vi "DrivetrainStateMachines(SubVI).vi"(4 "humanToSteady":bool, 5 "encoderSignalReceived?":bool, 6 "IMUtoSteady":bool, 7 "IMUSignalReceived?":bool, 9 "encoderToSteady":bool, 11 "humanSignalReceived?":bool) -> (3 "State Out":T1)   [LabVIEW 2017]
uses:
  Control 2.ctl
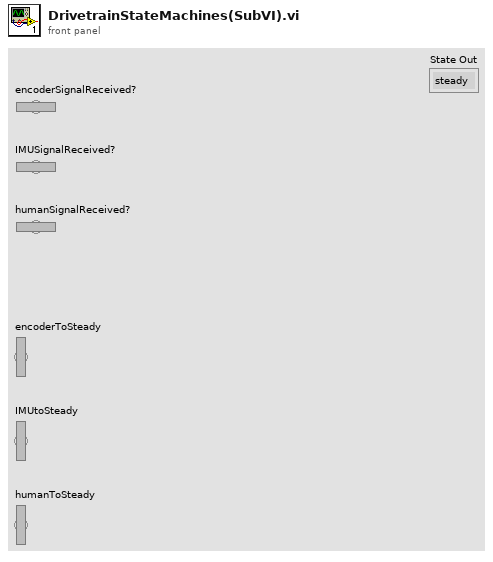
[diagram p1: front panel]
types:
  T1 = typedef "Control 2.ctl" = enum16{"steady", "driveByEncoder", "driveByIMU", "driveByHumans"}
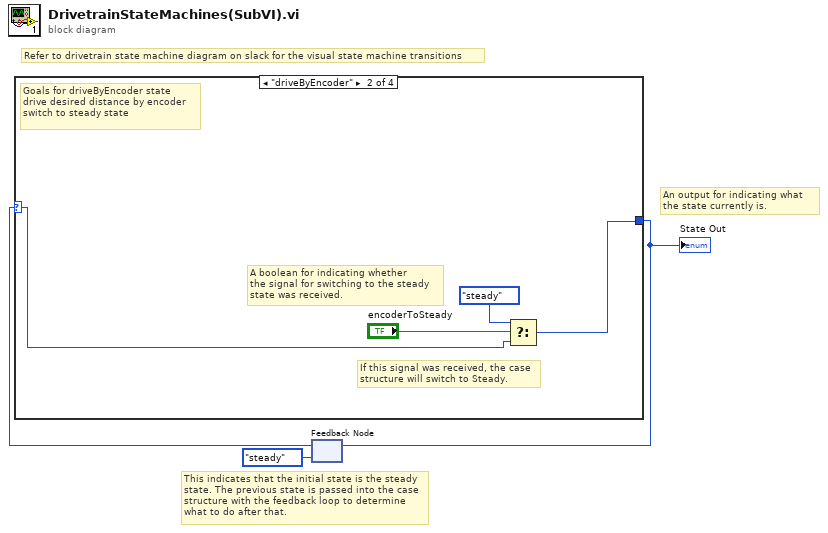
[diagram p0: block diagram]
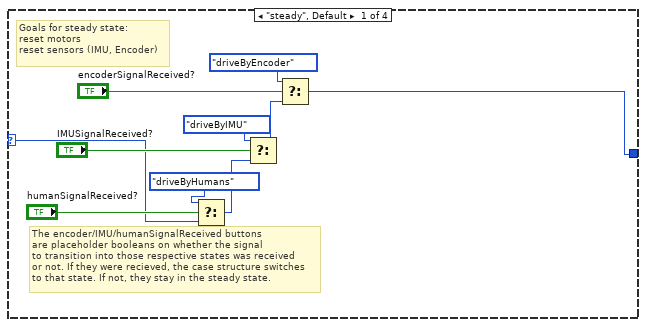
[diagram p2: hidden frame]
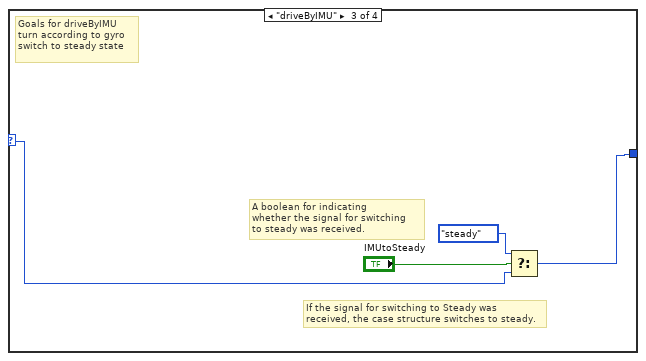
[diagram p3: hidden frame]
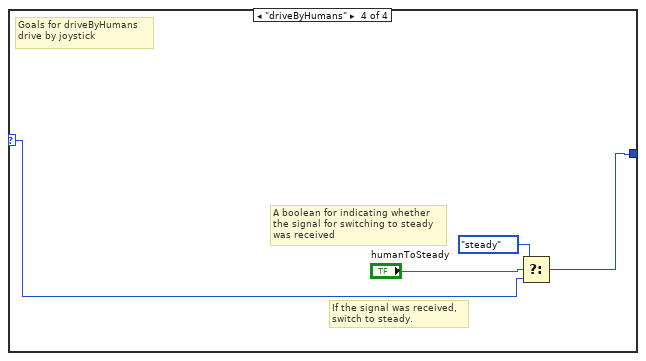
[diagram p4: hidden frame]
diagram:
  # "An output for indicating what\nthe state currently is."
  # "This indicates that the initial state is the steady\nstate. The previous state is passed into the case\nstructure with the feedback loop to determine\nwhat to do after that."
  # "Refer to drivetrain state machine diagram on slack for the visual state machine transitions"
  n1 = feedback #1(Control_2."steady") -> (w2:T1)
  n2 = case shown="\"driveByEncoder\"" w2 {
    selector: w2 -> [w4 w14 w18 w22]
    tunnel: [w7 w17 w20 w23] -> w3
    frame "steady", Default {
      # "The encoder/IMU/humanSignalReceived buttons\nare placeholder booleans on whether the signal\nto transition into those respective states was received\nor not. If they were recieved, the case structure switches\nto that state. If not, they stay in the steady state."
      # "Goals for steady state:\nreset motors\nreset sensors (IMU, Encoder)"
      n3 = Select(t=Control_2."driveByHumans", s="humanSignalReceived?", f=w4) -> (s? t:f=w6:T1)
      n4 = Select(t=Control_2."driveByIMU", s="IMUSignalReceived?", f=w6) -> (s? t:f=w5:T1)
      n5 = Select(t=Control_2."driveByEncoder", s="encoderSignalReceived?", f=w5) -> (s? t:f=w7:T1)
    }
    frame "driveByEncoder" {
      # "If this signal was received, the case\nstructure will switch to Steady."
      # "A boolean for indicating whether\nthe signal for switching to the steady\nstate was received."
      # "Goals for driveByEncoder state\ndrive desired distance by encoder\nswitch to steady state"
      n6 = Select(t=Control_2."steady", s="encoderToSteady", f=w14) -> (s? t:f=w17:T1)
    }
    frame "driveByIMU" {
      # "If the signal for switching to Steady was\nreceived, the case structure switches to steady."
      # "A boolean for indicating\nwhether the signal for switching \nto steady was received."
      # "Goals for driveByIMU\nturn according to gyro\nswitch to steady state"
      n7 = Select(t=Control_2."steady", s="IMUtoSteady", f=w18) -> (s? t:f=w20:T1)
    }
    frame "driveByHumans" {
      # "If the signal was received, \nswitch to steady."
      # "A boolean for indicating whether\nthe signal for switching to steady\nwas received"
      # "Goals for driveByHumans\ndrive by joystick"
      n8 = Select(t=Control_2."steady", s="humanToSteady", f=w22) -> (s? t:f=w23:T1)
    }
  }
  "State Out" <- w3
  n9 = feedback-in #1(w3) -> ()
